vi "Defaults.vi"(8 "error in (no error)":errorcluster, 11 "shell in":refnum<class "launcher.lvclass">) -> (0 "error out":errorcluster, 3 "shell out":refnum<class "launcher.lvclass">)   [LabVIEW 2021, in "launcher.lvclass"]
uses:
  launcher.lvclass
  C:/Program Files (x86)/National Instruments/LabVIEW 2021/user.lib/S2 Labs/Module Framework/Modules/Base/Module.lvclass
  <userlib>/S2 Labs/Module Framework/Modules/Logging/TypeDefs/_PARMS_.ctl
  <userlib>/S2 Labs/Logging Toolkit/TypeDefs/File Name Parms Cluster.ctl
  <userlib>/S2 Labs/Logging Toolkit/TDMS/TDMS.lvclass
  C:/Program Files (x86)/National Instruments/LabVIEW 2021/user.lib/S2 Labs/Logging Toolkit/Logging.lvclass
  <userlib>/S2 Labs/Logging Toolkit/TDMS/TDMS.lvclass/TDMS.ctl
  <userlib>/S2 Labs/Module Framework/Modules/Base/Module.lvclass/Module.ctl
  launcher.lvclass/launcher.ctl
  <userlib>/S2 Labs/Logging Toolkit/TDMS/Write BufferSize (Samples).vi
  <userlib>/S2 Labs/Module Framework/Modules/Base/Write Timeout (ms).vi
  <userlib>/S2 Labs/Module Framework/Modules/Base/Read App Directory.vi
  Accessors/Write ch_alias.vi
  Accessors/Write ch_units.vi
  Accessors/_Write Modules to Launch.vi
  <userlib>/S2 Labs/Module Framework/Modules/Logging/External Functions/Select TDMS.vi
  <userlib>/S2 Labs/Module Framework/Modules/Base/Module.lvclass
  <userlib>/S2 Labs/Module Framework/Modules/Logging/Logging Module.lvclass
  <userlib>/S2 Labs/Logging Toolkit/Logging.lvclass
  C:/Program Files (x86)/National Instruments/LabVIEW 2021/user.lib/S2 Labs/Logging Toolkit/TDMS/TDMS.lvclass
  <resource>/objmgr/nicontrollersysapi.rc
panel:
  out "By Type":T1(array[cluster])
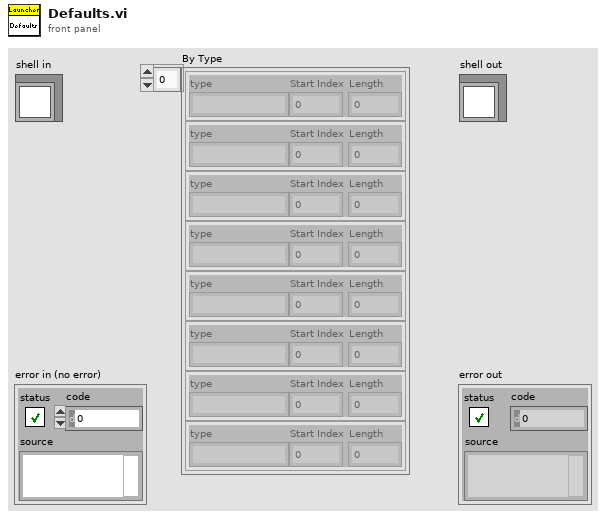
[diagram p1: front panel]
types:
  T1 = cluster{"type":string, "Start Index":i32, "Length":i32}[]
  T2 = cluster{"label":string, "alias":string, "unit":string}
  T3 = cluster{"label":string, "alias":string, "unit":string}[]
  T4 = typedef "Logging Module.lvclass/_PARMS_.ctl" = cluster{"Enabled?":bool, "Log Directory":path, "File Name Parms":T5, "Log Length (hrs)":dbl, "Max Storage Limit (MB)":dbl, "Max Storage Limit (Days)":dbl, "Defrag and Zip?":bool}
  T5 = typedef "Logging.lvclass/File Name Parms Cluster.ctl" = cluster{"Prefix":string, "Time Format":string, "Suffix":string, "Extension":string, "Create YYYY/MM subdirectories?":bool}
  T6 = typedef "Module.lvclass/Launch Module Typdef.ctl" = cluster{"Module":string, "Parameters":T7}
  T7 = typedef "Module.lvclass/Launch Module Parms.ctl" = cluster{"Name":string, "Arguments":string[], "Show FP?":bool}
  T8 = cluster{string, "chassis":cluster{"label":string, "alias":string, "unit":string}[]}
  T9 = cluster{string, "queues":cluster{"label":string, "alias":string, "unit":string}[]}
  T10 = cluster{string, "uptime":cluster{"label":string, "alias":string, "unit":string}[]}
  T11 = cluster{string, "memory":cluster{"label":string, "alias":string, "unit":string}[]}
  T12 = cluster{string, "storage":cluster{"label":string, "alias":string, "unit":string}[]}
  T13 = cluster{string, cluster{"label":string, "alias":string, "unit":string}[]}
  T14 = cluster{string, "storage":cluster{"label":string, "alias":string, "unit":string}[]}[]
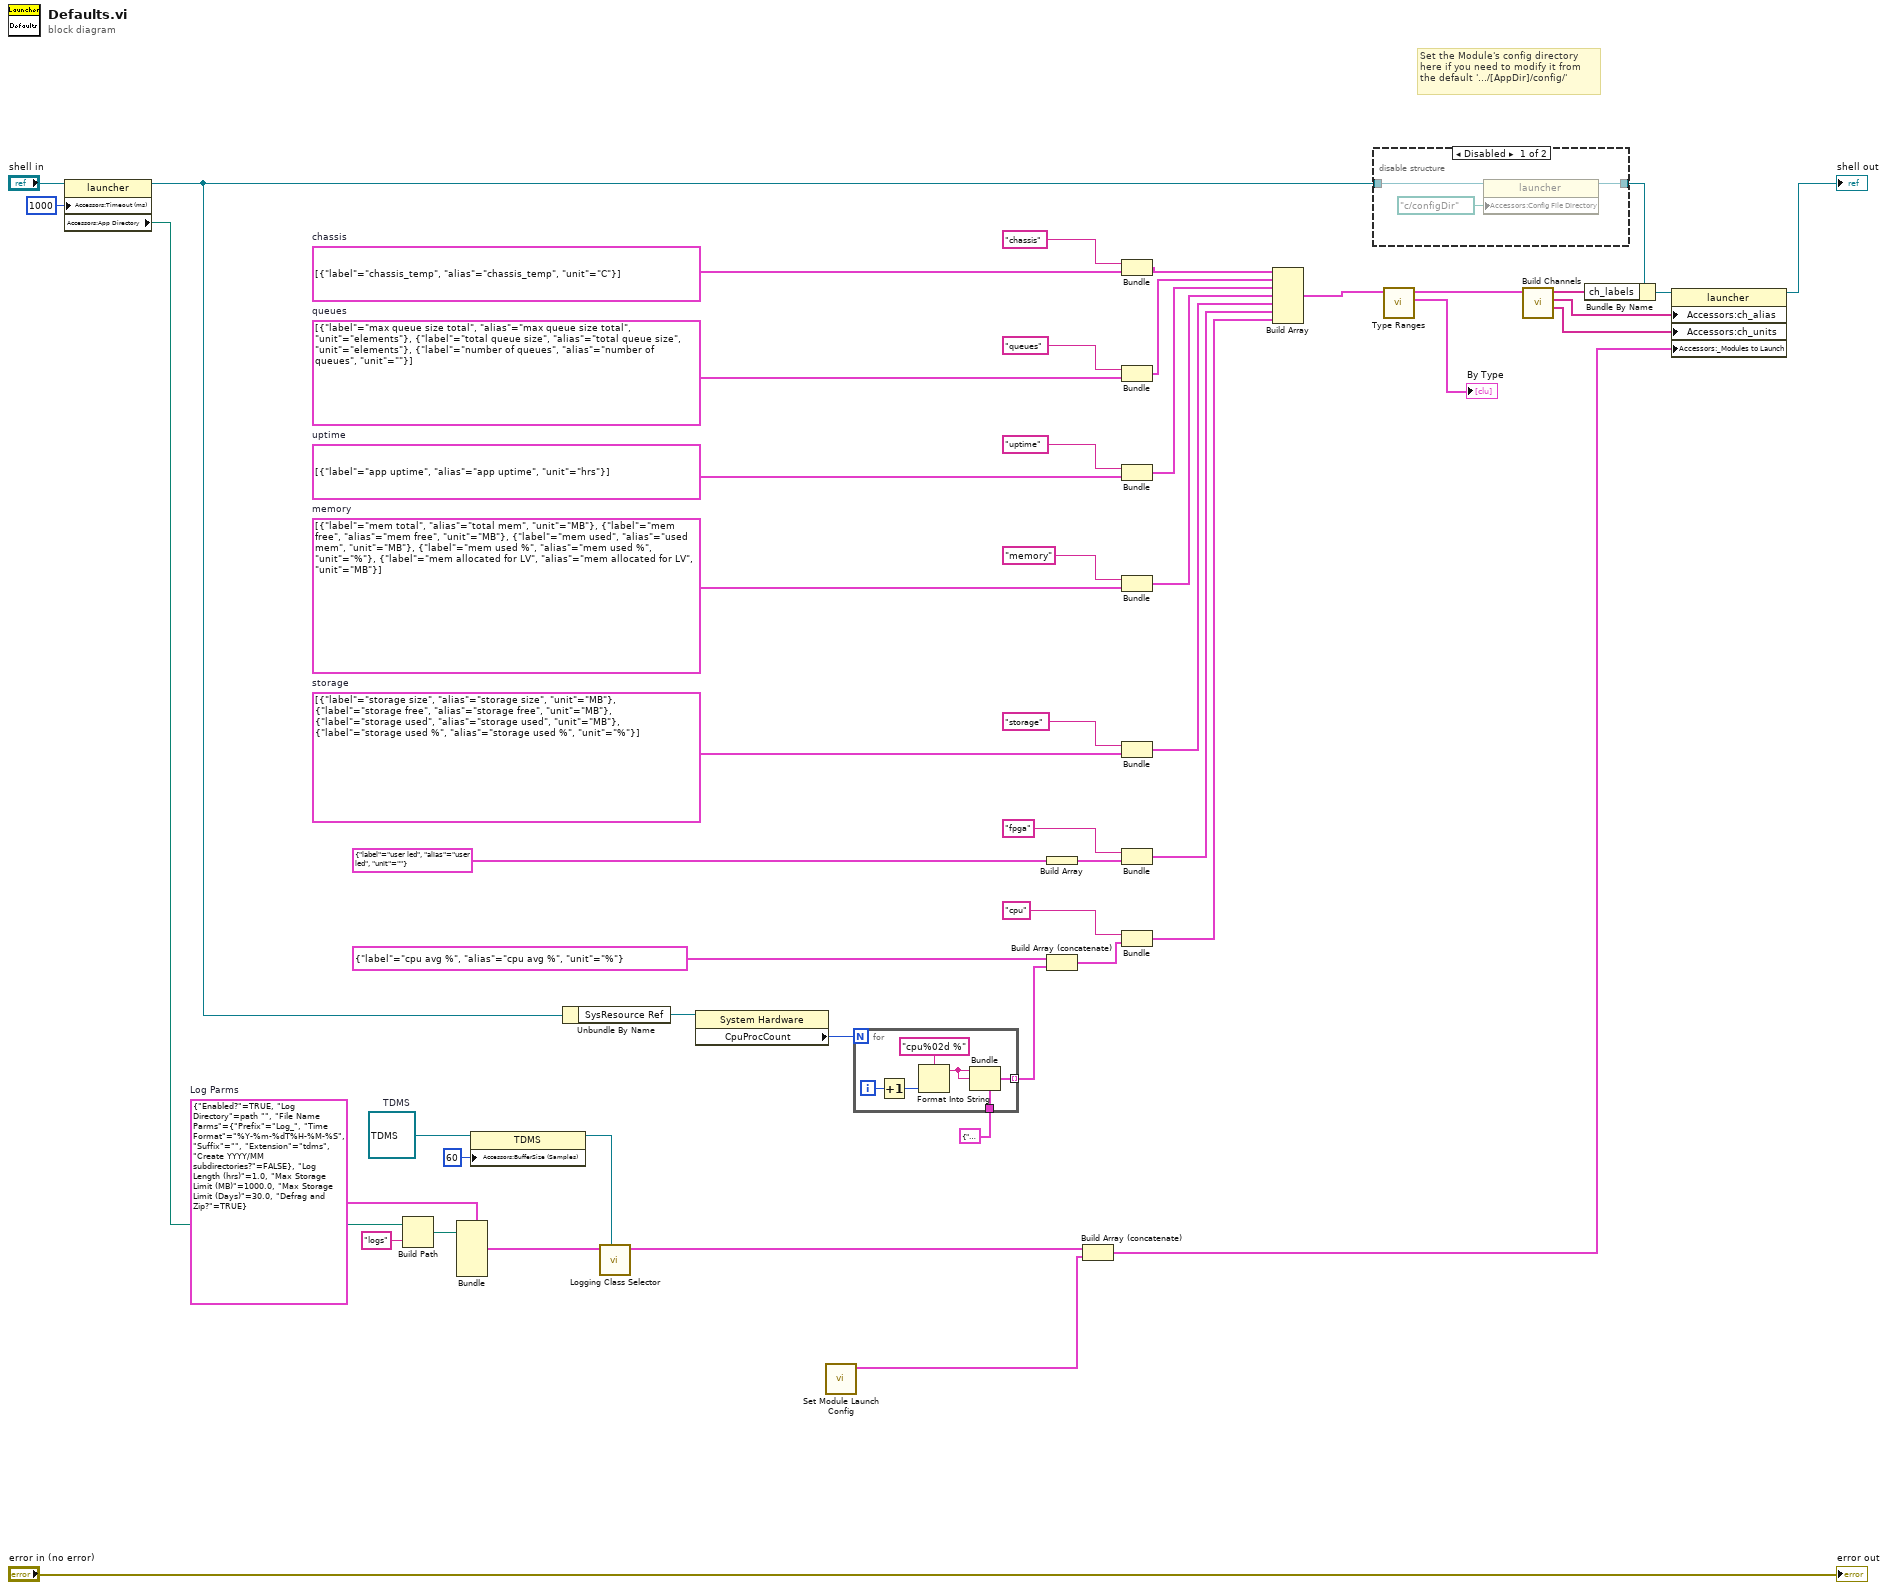
[diagram p0: block diagram]
diagram:
  w18 = refnum<class "TDMS.lvclass"> refnum  # TDMS
  w28 = T3 [{"label"="storage size", "alias"="storage size", "unit"="MB"}, {"label"="storage free", "alias"="storage free", "unit"="MB"}, {"label"="storage used", "alias"="storage used", "unit"="MB"}, {"label"="storage used %", "alias"="storage used %", "unit"="%"}]  # storage
  w29 = T3 [{"label"="mem total", "alias"="total mem", "unit"="MB"}, {"label"="mem free", "alias"="mem free", "unit"="MB"}, {"label"="mem used", "alias"="used mem", "unit"="MB"}, {"label"="mem used %", "alias"="mem used %", "unit"="%"}, {"label"="mem allocated for LV", "alias"="mem allocated for LV", "unit"="MB"}]  # memory
  w30 = T3 [{"label"="app uptime", "alias"="app uptime", "unit"="hrs"}]  # uptime
  w31 = T3 [{"label"="max queue size total", "alias"="max queue size total", "unit"="elements"}, {"label"="total queue size", "alias"="total queue size", "unit"="elements"}, {"label"="number of queues", "alias"="number of queues", "unit"=""}]  # queues
  w38 = T3 [{"label"="chassis_temp", "alias"="chassis_temp", "unit"="C"}]  # chassis
  w44 = T4 {"Enabled?"=TRUE, "Log Directory"=path "", "File Name Parms"={"Prefix"="Log_", "Time Format"="%Y-%m-%dT%H-%M-%S", "Suffix"="", "Extension"="tdms", "Create YYYY/MM subdirectories?"=FALSE}, "Log Length (hrs)"=1.0, "Max Storage Limit (MB)"=1000.0, "Max Storage Limit (Days)"=30.0, "Defrag and Zip?"=TRUE}  # Log Parms
  # "Set the Module's config directory\nhere if you need to modify it from\nthe default '.../[AppDir]/config/'"
  n1 = property class="launcher"(reference="shell in", "Accessors:Timeout (ms)"=1000 ("Module:Timeout (ms)")) -> (reference out=w14:refnum<class "launcher.lvclass">, "Accessors:App Directory"=w41:path)  [unwired: 1 in, 1 out]
  n2 = Build Path(base path=w41, name or relative path="logs") -> (appended path=w42:path)
  n3 = Bundle(cluster=w44, "Log Directory"=w42) -> (w43:T4)  [unwired: 6 in]
  n4 = property class="TDMS"(reference=w18, "Accessors:BufferSize (Samples)"=60 ("BufferSize (Samples)")) -> (reference out=w16:refnum<class "TDMS.lvclass">)  [unwired: 1 in, 1 out]
  n5 = Unbundle By Name(w14) -> ("SysResource Ref"=w13:refnum<k20>)
  n6 = call-poly <userlib>:"Logging Class Selector.vi"("Logging Class (TDMS)"=w16, "Log Parms"=w43) -> ("Launch Module Parms"=w45:T6)  [unwired: 9 in]
  n7 = property class="System Hardware"(reference=w13) -> ("CpuProcCount"=w12:i32)  [unwired: 1 in, 2 out]
  n8 = call "Set Module Launch Config.vi"() -> ("Modules to Launch"=w11:T6[])  [unwired: 11 in]
  n9 = for {
    N: w12 -> [_]
    tunnel: T2 {"label"="", "alias"="", "unit"="%"} ("ch") -> [w53]
    tunnel: [w52] -> w39 mode=indexing
    i -> [w57]
    n10 = Increment(x=w57) -> (x+1=w56:i32)
    n11 = Format Into String(format string="cpu%02d %", w56) -> (resulting string=w54:string)  [unwired: 2 in, 1 out]
    n12 = Bundle(cluster=w53, "label"=w54, "alias"=w54) -> (w52:T2)  [unwired: 1 in]
  }
  n13 = Build Array(T2 {"label"="user led", "alias"="user led", "unit"=""} ("ch")) -> (w5:T3)
  n14 = Build Array (concatenate)(T2 {"label"="cpu avg %", "alias"="cpu avg %", "unit"="%"} ("ch"), w39) -> (w27:T3)
  n15 = Build Array (concatenate)(w45, w11) -> (w8:T6[])
  n16 = Bundle("chassis", "chassis"=w38) -> (w26:T8)  [unwired: 1 in]
  n17 = Bundle("queues", "queues"=w31) -> (w25:T9)  [unwired: 1 in]
  n18 = Bundle("uptime", "uptime"=w30) -> (w24:T10)  [unwired: 1 in]
  n19 = Bundle("memory", "memory"=w29) -> (w23:T11)  [unwired: 1 in]
  n20 = Bundle("storage", "storage"=w28) -> (w22:T12)  [unwired: 1 in]
  n21 = Bundle("fpga", w5) -> (w1:T13)  [unwired: 1 in]
  n22 = Bundle("cpu", w27) -> (w2:T13)  [unwired: 1 in]
  n23 = Build Array(w26, w25, w24, w23, w22, w1, w2) -> (w21:T14)
  n24 = disable-structure shown="Disabled" {
    disable-tunnel: w14 -> [w60 w61]
    disable-tunnel: [w59 w61] -> w15
    frame Disabled {
      n25 = property class="launcher"(reference=w60, "Accessors:Config File Directory"=path "c:/configDir" ("Module:Config File Directory")) -> (reference out=w59:refnum<class "launcher.lvclass">)  [unwired: 1 in, 1 out]
    }
    frame Enabled {
    }
  }
  n26 = call <userlib>:"Type Ranges.vi"("Types"=w21) -> ("By Type"=→"By Type":T1, "channels"=w20:T3)  [unwired: 9 in]
  n27 = call <userlib>:"Build Channels.vi"("chs"=w20) -> ("ch_units"=w9:string[], "ch_alias"=w10:string[], "ch_labels"=w48:string[])  [unwired: 8 in]
  n28 = Bundle By Name(cluster=w15, "ch_labels"=w48) -> (w7:refnum<class "launcher.lvclass">)
  n29 = property class="launcher"(reference=w7, "Accessors:ch_alias"=w10, "Accessors:ch_units"=w9, "Accessors:_Modules to Launch"=w8) -> (reference out=→"shell out":refnum<class "launcher.lvclass">)  [unwired: 1 in, 1 out]
  "error out" <- "error in (no error)"
